vi "sensors and variables.vi"(11 "S P & V definitions":T3[](array[typedef]) {"value" format="%#_6p"; "variable"."Data average interval" min=0.0 format="%^#_3g"}) -> (0 "name (unit)":string[](array[string]), 1 "units":string[](array[string]), 2 "Variable names":string[](array[string]), 3 "Variable values":dbl[](array[numeric]), 4 "Calibrated data":T1 {"Sensor array"."scaled" format="%.2f"; "Sensor array"."voltage" format="%.4f"; "Time" format="%<%I:%M:%S%2u %p\n%m/%d/%Y>T"})   [LabVIEW 2015]
uses:
  variable setpoint.ctl
  data ave interval.ctl
  type specifier for control code.ctl
  TCP DAQ/Sensor data.ctl
  DAQ configuration/sensor cluster.ctl
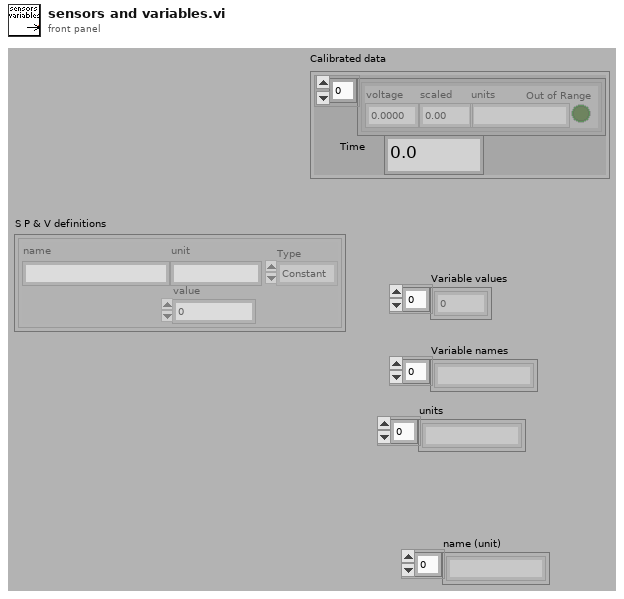
[diagram p1: front panel]
types:
  T1 = typedef "Sensor data.ctl" = cluster{" Sensor array":T2[], "Time":dbl}
  T2 = typedef "sensor cluster.ctl" = cluster{"voltage":sgl, "scaled":sgl, "units":string, "Out of Range":bool}
  T3 = typedef "variable setpoint.ctl" = cluster{"name":string, "unit":string, "value":dbl, "Type":enum16{"Constant", "Variable"}, "variable":cluster{"selected sensors":i32[], "selected set points":i32[], "VI":path, "Data average interval":T4, "code ref":T5}}
  T4 = typedef "data ave interval.ctl" = dbl
  T5 = typedef "type specifier for control code.ctl" = refnum<vi>
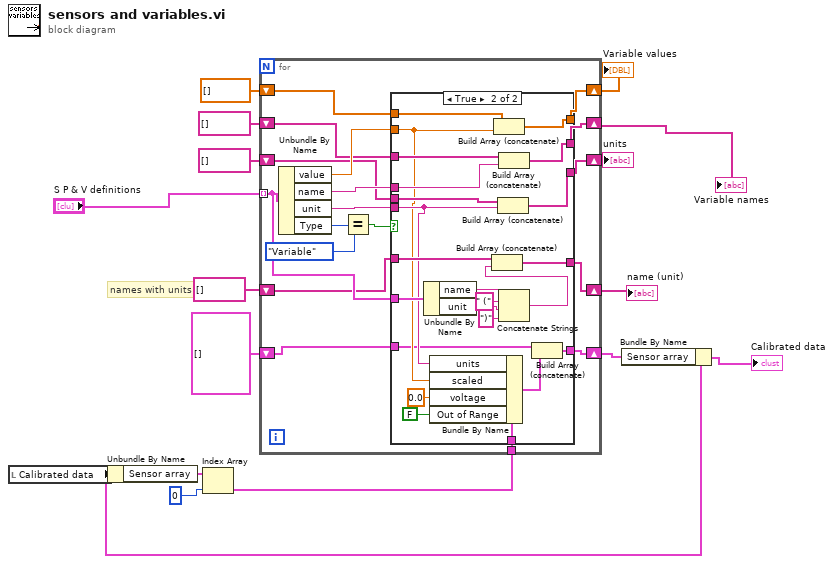
[diagram p0: block diagram]
diagram:
  # "names with units"
  n1 = local read "Calibrated data"() -> (w3:T1)
  n2 = Unbundle By Name(w3) -> ("Sensor array"=w7:T2[])
  n3 = Index Array(array=w7, index=0) -> (element=w4:T2)
  n4 = for {
    tunnel: "S P & V definitions" -> [w22] mode=indexing
    shift-right: [w31] -> w12
    shift-left: string[] [] -> [w24]
    shift-right: [w28] -> w13
    shift-left: dbl[] [] -> [w29]
    shift-right: [w25] -> w10
    shift-left: string[] [] -> [w23]
    shift-right: [w20] -> w8
    shift-left: string[] [] -> [w21]
    shift-right: [w18] -> w2
    shift-left: T2[] [] -> [w17]
    tunnel: w4 -> [w19]
    n5 = Unbundle By Name(w22) -> ("value"=w30:dbl, "name"=w32:string, "unit"=w26:string, "Type"=w27:enum16{"Constant", "Variable"})
    n6 = Equal?(x=w27, y=enum16{"Constant", "Variable"}."Variable" ("Type")) -> (x = y?=w33:bool)
    n7 = case shown="True" w33 {
      tunnel: w32 -> [_ w58]
      tunnel: w24 -> [w39 w62]
      tunnel: [w39 w61] -> w31
      tunnel: w30 -> [_ w45]
      tunnel: w29 -> [w38 w60]
      tunnel: [w38 w59] -> w28
      tunnel: w26 -> [_ w46]
      tunnel: [w37 w57] -> w25
      tunnel: w23 -> [w37 w56]
      tunnel: w22 -> [_ w53]
      tunnel: w21 -> [w36 w50]
      tunnel: [w36 w49] -> w20
      tunnel: w19 -> [_ w44]
      tunnel: [w35 w41] -> w18
      tunnel: w17 -> [w35 w40]
      frame False {
      }
      frame True {
        n8 = Unbundle By Name(w53) -> ("name"=w52:string, "unit"=w55:string)
        n9 = Bundle By Name(cluster=w44, "units"=w46, "scaled"=w45, "voltage"=sgl 0.0, "Out of Range"=FALSE) -> (w42:T2)
        n10 = Build Array (concatenate)(w60, w45) -> (w59:dbl[])
        n11 = Build Array (concatenate)(w56, w46) -> (w57:string[])
        n12 = Build Array (concatenate)(w62, w58) -> (w61:string[])
        n13 = Concatenate Strings(w52, " (" ("string"), w55, ")" ("string")) -> (w51:string)
        n14 = Build Array (concatenate)(w50, w51) -> (w49:string[])
        n15 = Build Array (concatenate)(w40, w42) -> (w41:T2[])
      }
    }
  }
  "Variable names" <- w12
  "Variable values" <- w13
  "units" <- w10
  "name (unit)" <- w8
  n16 = Bundle By Name(cluster=w3, "Sensor array"=w2) -> (→"Calibrated data":T1)
